vi "CCE MGLD PMJD PF SubVI01.vi"(11 "captura":T1) -> (0 "Image 4":T1(plugin-control), 1 "y":sgl, 2 "x":sgl, 3 "tapa detectada":bool)   [LabVIEW 2020]
uses:
  <vilib>/vision/Image Controls.llb/IMAQ Image.ctl
  <vilib>/vision/NI_Vision_Development_Module.lvlib
panel:
  in  "File Path":path=path "C:/Users/kitsu/Documents/SVA/proyecto final/tapa.png"
  out "Image 2":T1(plugin-control)
  out "patron":T1(plugin-control)
  out "Matches (real-world)":T2(array[cluster]) {"Bounding Box"."y" format="%.2f"; "Bounding Box"."x" format="%.2f"; "Score" format="%.2f"; "Scale" format="%.2f"; "Angle" format="%.2f"; "Position"."y" format="%.2f"; "Position"."x" format="%.2f"}
  out "Number of Matches":i32
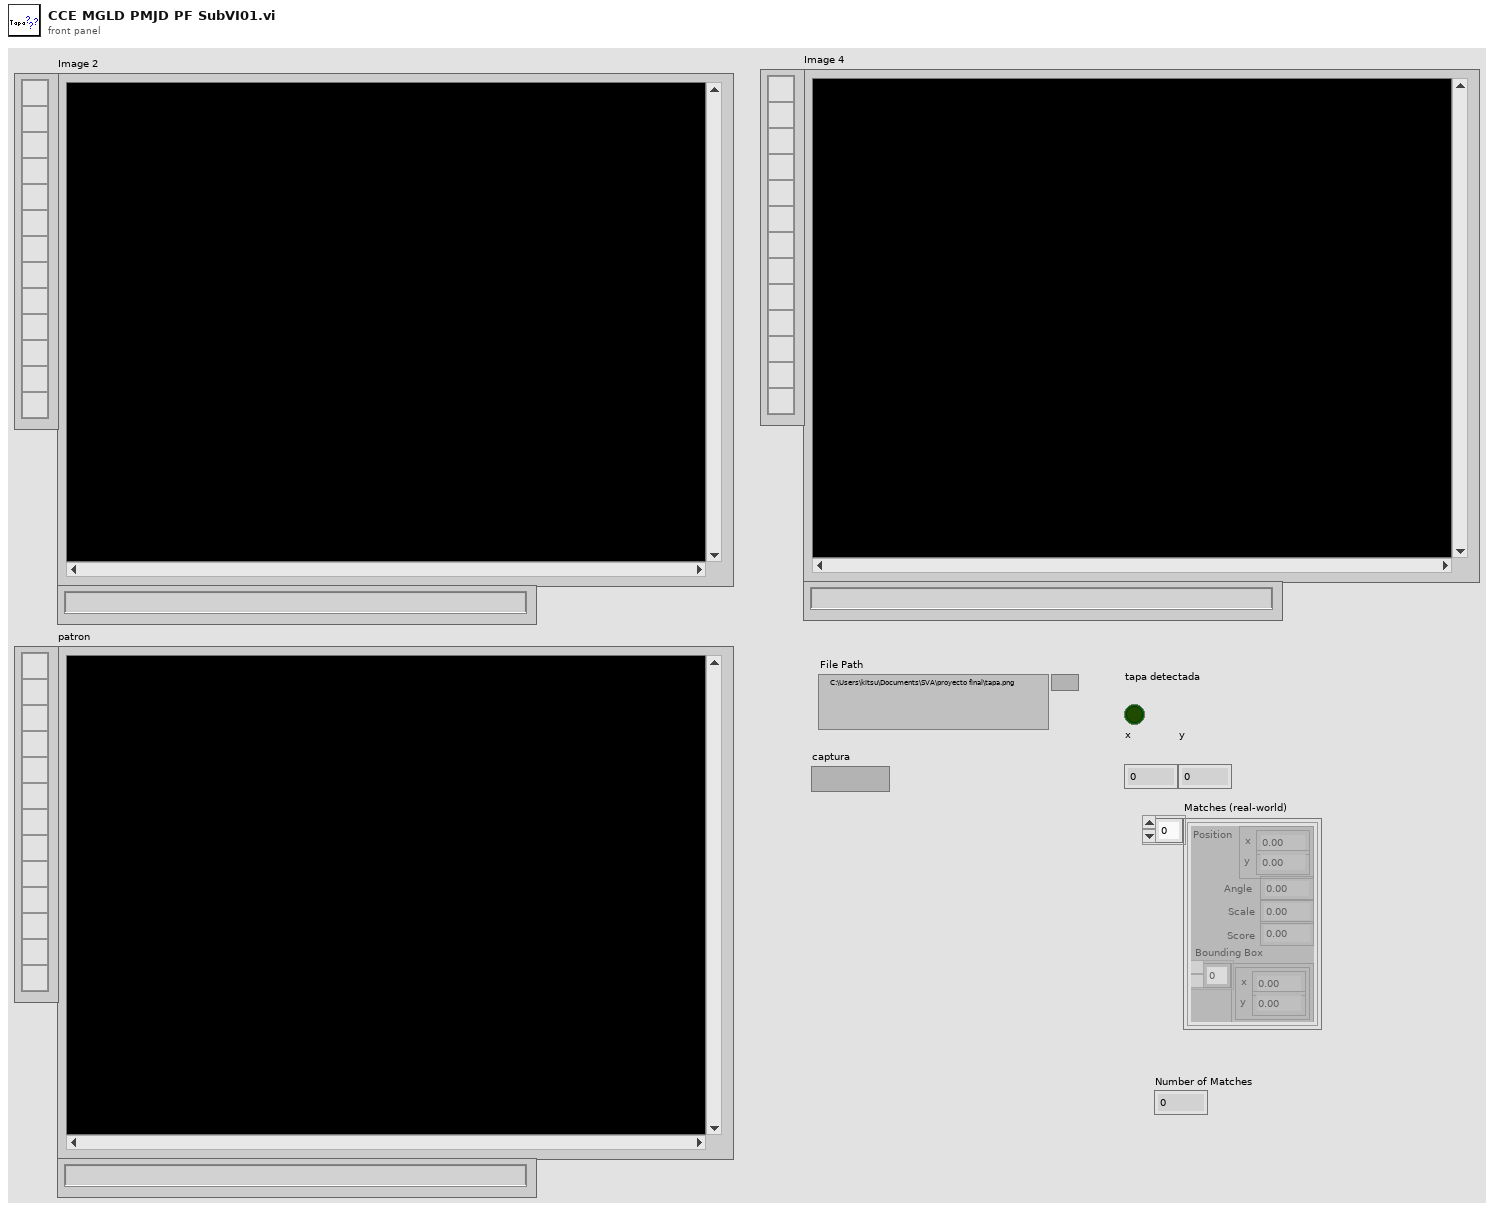
[diagram p1: front panel]
types:
  T1 = typedef "IMAQ Image.ctl" = refnum<image>
  T2 = cluster{"Position":cluster{"x":sgl, "y":sgl}, "Angle":sgl, "Scale":sgl, "Score":sgl, "Bounding Box":cluster{"x":sgl, "y":sgl}[]}[]
  T3 = cluster{"Number of Matches Requested":i32, "Minimum Match Score":sgl, "Angle Ranges":cluster{"Start Angle":sgl, "End Angle":sgl}[]}
  T4 = typedef "Image Type" = u32
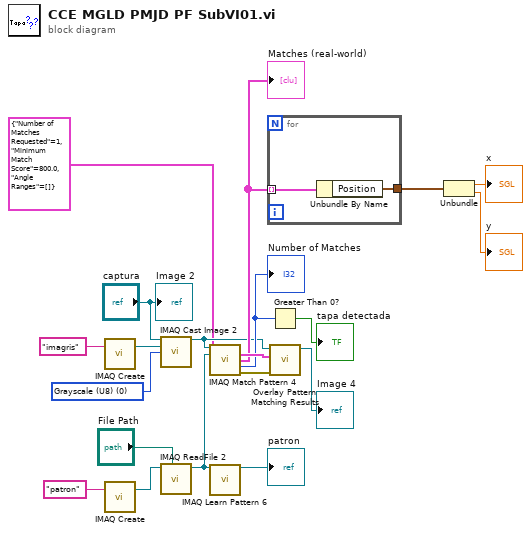
[diagram p0: block diagram]
diagram:
  w10 = T4 0 items=["Grayscale (U8)", "Grayscale (I16)", "Grayscale (SGL)", "Complex (CSG)", "RGB (U32)", "HSL (U32)", "RGB (U64)", "Grayscale (U16)"] ("Image Type")
  n1 = call "IMAQ Create"("Image Name"="imagris") -> ("New Image"=w15:T1)  [unwired: 4 in, 1 out]
  n2 = call "IMAQ Create"("Image Name"="patron") -> ("New Image"=w17:T1)  [unwired: 4 in, 1 out]
  n3 = call "IMAQ Cast Image 2"("Image Src"="captura", "Image Dst"=w15, "Image Type"=w10) -> ("Image Dst Out"=w2:T1)  [unwired: 11 in, 1 out]
  n4 = call "IMAQ ReadFile 2"("File Path"="File Path", "Image"=w17) -> ("Image Out"=w16:T1)  [unwired: 5 in, 4 out]
  n5 = call "IMAQ Match Pattern 4"("Image"=w2, "Template Image"=w16, "Parameters"=T3 {"Number of Matches Requested"=1, "Minimum Match Score"=800.0, "Angle Ranges"=[]}) -> ("Matches (pixel)"=w13:T2, "Matches (real-world)"=w9:T2, "Number of Matches"=w8:i32, "error out"=w12:errorcluster)  [unwired: 8 in, 1 out]
  "Matches (real-world)" <- w9
  "Number of Matches" <- w8
  n6 = call "IMAQ Learn Pattern 6"("Image"=w16) -> ("Template Image Out"=→"patron":T1)  [unwired: 12 in, 2 out]
  n7 = for {
    tunnel: w9 -> [w22] mode=indexing
    tunnel: [w21] -> w6
    n8 = Unbundle By Name(w22) -> ("Position"=w21:cluster{"x":sgl, "y":sgl})
  }
  n9 = Greater Than 0?(x=w8) -> (x > 0?=→"tapa detectada":bool)
  n10 = call "Overlay Pattern Matching Results.vi"("error in"=w12, "Matches"=w13, "Image"=w2) -> ("Image Out"=→"Image 4":T1)  [unwired: 7 in, 1 out]
  n11 = Unbundle(w6) -> ("x"=→"x":sgl, "y"=→"y":sgl)
  "Image 2" <- "captura"
